vi "New Equalizer Code.vi"(11 "Reference":cdb[](array[numeric])) -> (3 "Hest":cdb[](array[numeric]))   [LabVIEW 2012]
doc: "Estimates channel based on received refrence symbols and known refrecnce symbols"
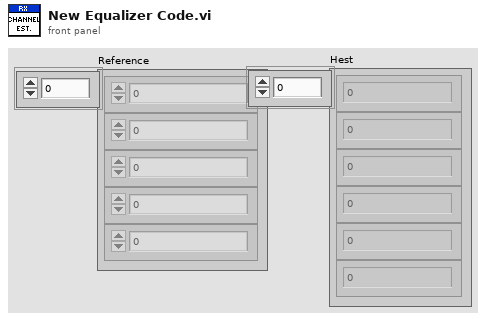
[diagram p1: front panel]
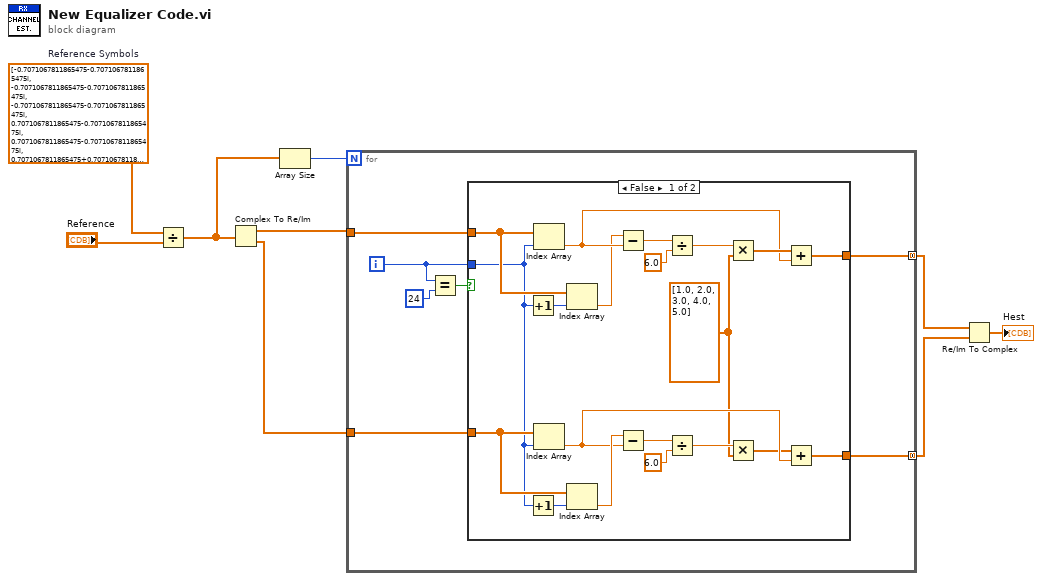
[diagram p0: block diagram]
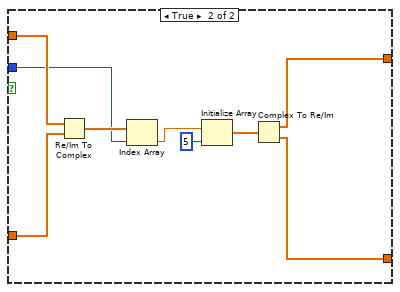
[diagram p2: hidden frame]
diagram:
  w6 = cdb[] [-0.7071067811865475-0.7071067811865475i, -0.7071067811865475-0.7071067811865475i, -0.7071067811865475-0.7071067811865475i, 0.7071067811865475-0.7071067811865475i, 0.7071067811865475-0.7071067811865475i, 0.7071067811865475+0.7071067811865475i, 0.7071067811865475-0.7071067811865475i, -0.7071067811865475-0.7071067811865475i, 0.7071067811865475+0.7071067811865475i, -0.7071067811865475+0.7071067811865475i, -0.7071067811865475-0.7071067811865475i, -0.7071067811865475+0.7071067811865475i, -0.7071067811865475+0.7071067811865475i, 0.7071067811865475-0.7071067811865475i, -0.7071067811865475+0.7071067811865475i, -0.7071067811865475+0.7071067811865475i, 0.7071067811865475-0.7071067811865475i, -0.7071067811865475+0.7071067811865475i, -0.7071067811865475-0.7071067811865475i, 0.7071067811865475-0.7071067811865475i, 0.7071067811865475+0.7071067811865475i, -0.7071067811865475-0.7071067811865475i, -0.7071067811865475-0.7071067811865475i, 0.7071067811865475-0.7071067811865475i, -0.7071067811865475-0.7071067811865475i, 0.7071067811865475-0.7071067811865475i, 0.7071067811865475-0.7071067811865475i, 0.7071067811865475+0.7071067811865475i, 0.7071067811865475+0.7071067811865475i, -0.7071067811865475-0.7071067811865475i, -0.7071067811865475+0.7071067811865475i, -0.7071067811865475+0.7071067811865475i, 0.7071067811865475-0.7071067811865475i, -0.7071067811865475-0.7071067811865475i, -0.7071067811865475+0.7071067811865475i, -0.7071067811865475-0.7071067811865475i, -0.7071067811865475+0.7071067811865475i, 0.7071067811865475-0.7071067811865475i, 0.7071067811865475+0.7071067811865475i, 0.7071067811865475+0.7071067811865475i, 0.7071067811865475-0.7071067811865475i, -0.7071067811865475-0.7071067811865475i, -0.7071067811865475+0.7071067811865475i, -0.7071067811865475+0.7071067811865475i, -0.7071067811865475-0.7071067811865475i, -0.7071067811865475-0.7071067811865475i, -0.7071067811865475+0.7071067811865475i, -0.7071067811865475+0.7071067811865475i, -0.7071067811865475+0.7071067811865475i, -0.7071067811865475+0.7071067811865475i]  # Reference Symbols
  n1 = Divide(x=w6, y="Reference") -> (x/y=w1:cdb[])
  n2 = Complex To Re/Im(x + iy=w1) -> (x=w8:dbl[], y=w7:dbl[])
  n3 = Array Size(array=w1) -> (size(s)=w9:i32)
  n4 = for {
    N: w9 -> [_]
    tunnel: [w14] -> w4 mode=concatenating
    tunnel: w8 -> [w10]
    tunnel: w7 -> [w16]
    tunnel: [w13] -> w3 mode=concatenating
    i -> [w12]
    n5 = Equal?(x=w12, y=24) -> (x = y?=w11:bool)
    n6 = case shown="False" w11 {
      tunnel: w10 -> [w29 w45]
      tunnel: w16 -> [w21 w44]
      tunnel: [w19 w38] -> w14
      tunnel: [w18 w37] -> w13
      tunnel: w12 -> [w17 w42]
      frame False {
        w20 = dbl[] [1.0, 2.0, 3.0, 4.0, 5.0]
        n7 = Increment(x=w17) -> (x+1=w36:i32)
        n8 = Increment(x=w17) -> (x+1=w22:i32)
        n9 = Index Array(array=w29, index=w17) -> (element=w31:dbl)
        n10 = Index Array(array=w21, index=w17) -> (element=w27:dbl)
        n11 = Index Array(array=w29, index=w36) -> (element=w30:dbl)
        n12 = Index Array(array=w21, index=w22) -> (element=w28:dbl)
        n13 = Subtract(x=w30, y=w31) -> (x-y=w35:dbl)
        n14 = Subtract(x=w28, y=w27) -> (x-y=w23:dbl)
        n15 = Divide(x=w35, y=6.0) -> (x/y=w33:dbl)
        n16 = Divide(x=w23, y=6.0) -> (x/y=w25:dbl)
        n17 = Multiply(x=w33, y=w20) -> (x*y=w32:dbl[])
        n18 = Multiply(x=w25, y=w20) -> (x*y=w26:dbl[])
        n19 = Add(x=w32, y=w31) -> (x+y=w19:dbl[])
        n20 = Add(x=w26, y=w27) -> (x+y=w18:dbl[])
      }
      frame True {
        n21 = Re/Im To Complex(1:w44, 2:w45) -> (0:w43:cdb[])
        n22 = Index Array(array=w43, index=w42) -> (element=w41:cdb)
        n23 = Initialize Array(w41, 5 ("dimension size")) -> (w39:cdb[])
        n24 = Complex To Re/Im(x + iy=w39) -> (x=w38:dbl[], y=w37:dbl[])
      }
    }
  }
  n25 = Re/Im To Complex(1:w3, 2:w4) -> (0:→"Hest":cdb[])
